vi "sub_tabelle_loeschen.vi"(1 "Numerisches Element":i32, 2 "Array":string[][](array[string])) -> ()   [LabVIEW 2009]
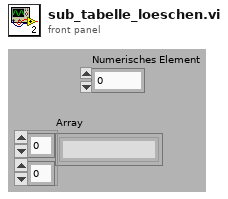
[diagram p1: front panel]
types:
  T1 = enum16{"open", "replace", "create", "open or create", "replace or create", "replace or create with confirmation"}
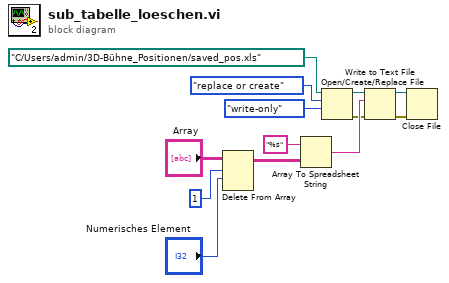
[diagram p0: block diagram]
diagram:
  n1 = Delete From Array(array="Array", length=1 ("Länge"), index (row)="Numerisches Element") -> (array with subset deleted=w13:string[][])  [unwired: 1 in, 1 out]
  n2 = Array To Spreadsheet String(array=w13, 3:"%s" ("Format-String")) -> (spreadsheet string=w12:string)  [unwired: 1 in]
  n3 = Open/Create/Replace File(file path (use dialog)=path "C:/Users/admin/3D-Bühne_Positionen/saved_pos.xls" ("Dateipfad (Dialog verwenden)"), operation (0:open)=T1."replace or create" ("Operation (0:Öffnen)"), access (0:read/write)=enum16{"read/write", "read-only", "write-only"}."write-only" ("Zugriff (0:Lesen/Schreiben)")) -> (refnum out=w5:refnum<file>, error out=w1:errorcluster)  [unwired: 3 in, 1 out]
  n4 = Write to Text File(file (use dialog)=w5, text=w12, error in=w1) -> (refnum out=w7:refnum<file>, error out=w8:errorcluster)  [unwired: 1 in, 1 out]
  n5 = Close File(refnum=w7, error in=w8) -> ()  [unwired: 2 out]
